vi "60_cm_Scoring.vi"() -> (0 "String":string, 3 "Cluster":cluster{"State":T1, "Drive Control":T2}={"State"=enum."Stop", "Drive Control"={"Left X"=0, "Left Y"=0, "Right Y"=0, "Power (100)"=0, "Wait (ms)"=0, "Enc/Deg Target"=0, "Move Type"=enum."Relative Degrees"}} {"Drive Control"."Power (100)" min=-100 max=100})   [LabVIEW 2012, in "Serenity_mk2.lvrbt"]
uses:
  Serenity_mk2.lvrbt
  State_Typ.ctl
  auto_drive_TYP.ctl
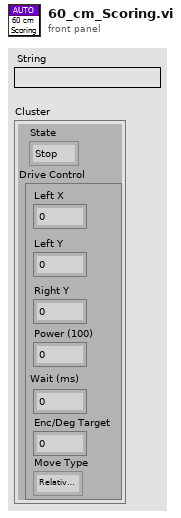
[diagram p1: front panel]
types:
  T1 = typedef "State_Typ.ctl" = enum16{"Sweeper", "Stop", "Check for Position 3", "Check for Position 2", "Move", "Reset Enc", "Read Enc", "Lift", "Dump Close"}
  T2 = typedef "auto_drive_TYP.ctl" = cluster{"Left X":i8, "Left Y":i8, "Right Y":i8, "Power (100)":i8, "Wait (ms)":u32, "Enc/Deg Target":i32, "Move Type":enum16{"Relative Degrees", "Wait", "Encoder"}}
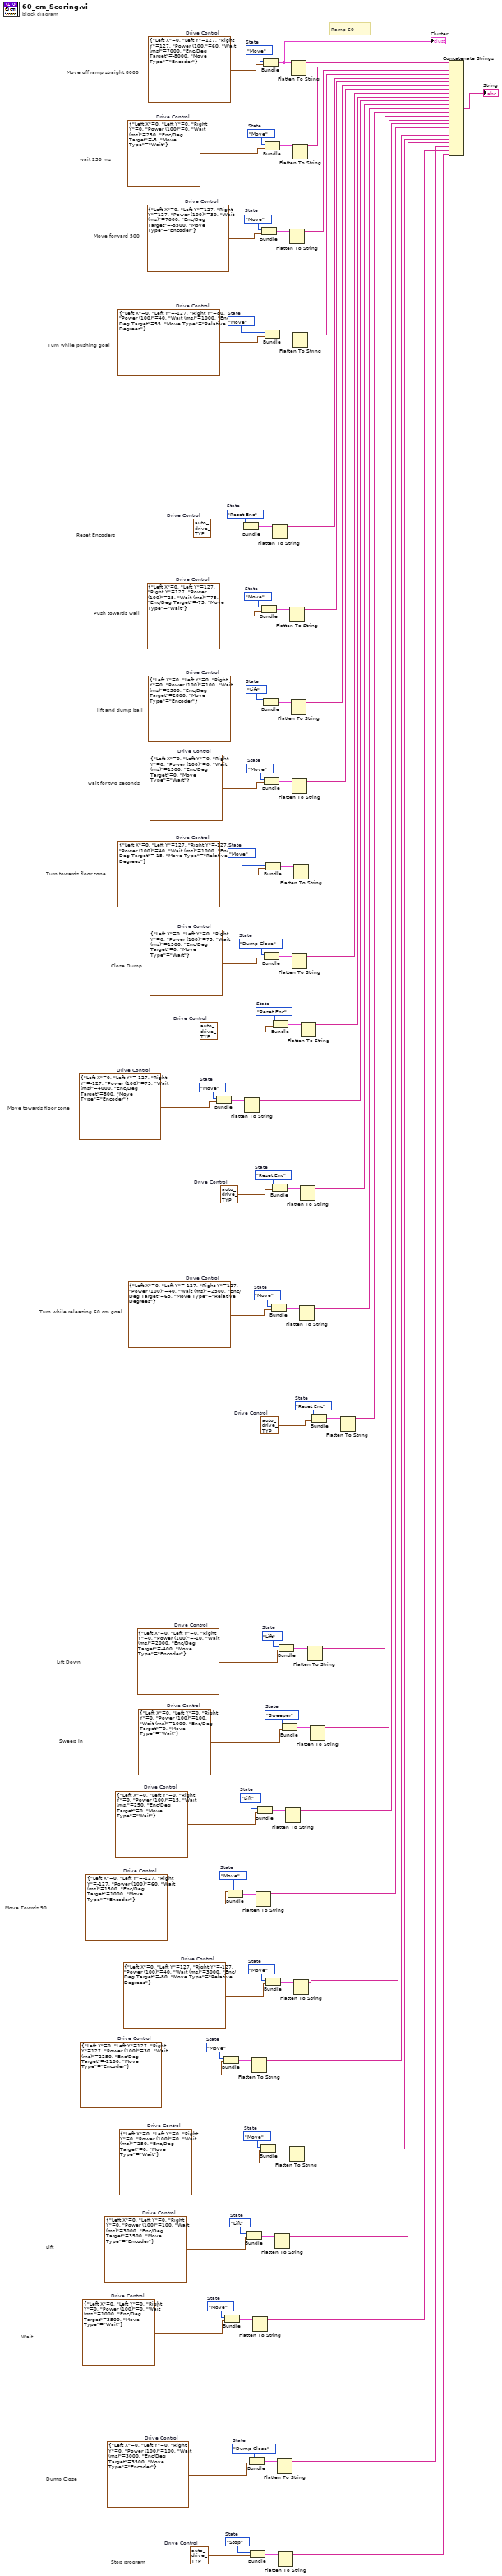
[diagram p0: block diagram]
diagram:
  w5 = T2 {"Left X"=0, "Left Y"=0, "Right Y"=0, "Power (100)"=0, "Wait (ms)"=1000, "Enc/Deg Target"=3500, "Move Type"=enum."Wait"}  # Drive Control
  w3 = State_Typ."Move"  # State
  w8 = T2 {"Left X"=0, "Left Y"=0, "Right Y"=0, "Power (100)"=100, "Wait (ms)"=3000, "Enc/Deg Target"=3500, "Move Type"=enum."Encoder"}  # Drive Control
  w6 = State_Typ."Dump Close"  # State
  w13 = T2 {"Left X"=0, "Left Y"=0, "Right Y"=0, "Power (100)"=100, "Wait (ms)"=3000, "Enc/Deg Target"=3500, "Move Type"=enum."Encoder"}  # Drive Control
  w11 = State_Typ."Lift"  # State
  w16 = T2 {"Left X"=0, "Left Y"=0, "Right Y"=0, "Power (100)"=0, "Wait (ms)"=250, "Enc/Deg Target"=0, "Move Type"=enum."Wait"}  # Drive Control
  w14 = State_Typ."Move"  # State
  w18 = T2 {"Left X"=0, "Left Y"=-127, "Right Y"=50, "Power (100)"=40, "Wait (ms)"=650, "Enc/Deg Target"=-6500, "Move Type"=enum."Wait"}  # Drive Control
  w19 = State_Typ."Reset Enc"  # State
  w27 = T2 {"Left X"=0, "Left Y"=0, "Right Y"=0, "Power (100)"=15, "Wait (ms)"=250, "Enc/Deg Target"=0, "Move Type"=enum."Wait"}  # Drive Control
  w25 = State_Typ."Lift"  # State
  w32 = T2 {"Left X"=0, "Left Y"=0, "Right Y"=0, "Power (100)"=-10, "Wait (ms)"=2000, "Enc/Deg Target"=-400, "Move Type"=enum."Encoder"}  # Drive Control
  w30 = State_Typ."Lift"  # State
  w35 = T2 {"Left X"=0, "Left Y"=0, "Right Y"=0, "Power (100)"=100, "Wait (ms)"=1000, "Enc/Deg Target"=0, "Move Type"=enum."Wait"}  # Drive Control
  w33 = State_Typ."Sweeper"  # State
  w38 = T2 {"Left X"=0, "Left Y"=-127, "Right Y"=-127, "Power (100)"=60, "Wait (ms)"=1500, "Enc/Deg Target"=1000, "Move Type"=enum."Encoder"}  # Drive Control
  w36 = State_Typ."Move"  # State
  w41 = T2 {"Left X"=0, "Left Y"=127, "Right Y"=-127, "Power (100)"=40, "Wait (ms)"=3000, "Enc/Deg Target"=-80, "Move Type"=enum."Relative Degrees"}  # Drive Control
  w39 = State_Typ."Move"  # State
  w46 = T2 {"Left X"=0, "Left Y"=127, "Right Y"=127, "Power (100)"=30, "Wait (ms)"=2250, "Enc/Deg Target"=-2100, "Move Type"=enum."Encoder"}  # Drive Control
  w44 = State_Typ."Move"  # State
  w51 = T2 {"Left X"=0, "Left Y"=127, "Right Y"=127, "Power (100)"=20, "Wait (ms)"=7000, "Enc/Deg Target"=-8500, "Move Type"=enum."Encoder"}  # Drive Control
  w50 = State_Typ."Reset Enc"  # State
  w54 = T2 {"Left X"=0, "Left Y"=127, "Right Y"=127, "Power (100)"=25, "Wait (ms)"=75, "Enc/Deg Target"=-75, "Move Type"=enum."Wait"}  # Drive Control
  w53 = State_Typ."Move"  # State
  w58 = T2 {"Left X"=0, "Left Y"=0, "Right Y"=0, "Power (100)"=50, "Wait (ms)"=4000, "Enc/Deg Target"=-9000, "Move Type"=enum."Encoder"}  # Drive Control
  w59 = State_Typ."Reset Enc"  # State
  w61 = T2 {"Left X"=0, "Left Y"=-127, "Right Y"=-127, "Power (100)"=75, "Wait (ms)"=4000, "Enc/Deg Target"=800, "Move Type"=enum."Encoder"}  # Drive Control
  w62 = State_Typ."Move"  # State
  w65 = T2 {"Left X"=0, "Left Y"=-127, "Right Y"=80, "Power (100)"=40, "Wait (ms)"=1000, "Enc/Deg Target"=55, "Move Type"=enum."Relative Degrees"}  # Drive Control
  w66 = State_Typ."Move"  # State
  w69 = T2 {"Left X"=0, "Left Y"=0, "Right Y"=0, "Power (100)"=0, "Wait (ms)"=250, "Enc/Deg Target"=-5, "Move Type"=enum."Wait"}  # Drive Control
  w70 = State_Typ."Move"  # State
  w73 = T2 {"Left X"=0, "Left Y"=127, "Right Y"=127, "Power (100)"=30, "Wait (ms)"=7000, "Enc/Deg Target"=-8500, "Move Type"=enum."Encoder"}  # Drive Control
  w74 = State_Typ."Move"  # State
  w78 = T2 {"Left X"=0, "Left Y"=0, "Right Y"=0, "Power (100)"=75, "Wait (ms)"=1500, "Enc/Deg Target"=0, "Move Type"=enum."Wait"}  # Drive Control
  w79 = State_Typ."Dump Close"  # State
  w101 = T2 {"Left X"=0, "Left Y"=0, "Right Y"=0, "Power (100)"=0, "Wait (ms)"=1500, "Enc/Deg Target"=0, "Move Type"=enum."Wait"}  # Drive Control
  w102 = State_Typ."Move"  # State
  w98 = T2 {"Left X"=0, "Left Y"=-127, "Right Y"=50, "Power (100)"=40, "Wait (ms)"=650, "Enc/Deg Target"=-6500, "Move Type"=enum."Wait"}  # Drive Control
  w99 = State_Typ."Reset Enc"  # State
  w95 = T2 {"Left X"=0, "Left Y"=-127, "Right Y"=127, "Power (100)"=40, "Wait (ms)"=2500, "Enc/Deg Target"=65, "Move Type"=enum."Relative Degrees"}  # Drive Control
  w96 = State_Typ."Move"  # State
  w85 = T2 {"Left X"=0, "Left Y"=0, "Right Y"=-127, "Power (100)"=40, "Wait (ms)"=700, "Enc/Deg Target"=-6500, "Move Type"=enum."Wait"}  # Drive Control
  w92 = T2 {"Left X"=0, "Left Y"=127, "Right Y"=-127, "Power (100)"=40, "Wait (ms)"=1000, "Enc/Deg Target"=-15, "Move Type"=enum."Relative Degrees"}  # Drive Control
  w93 = State_Typ."Move"  # State
  w90 = T2 {"Left X"=0, "Left Y"=0, "Right Y"=0, "Power (100)"=100, "Wait (ms)"=2500, "Enc/Deg Target"=2800, "Move Type"=enum."Encoder"}  # Drive Control
  w89 = State_Typ."Lift"  # State
  w86 = State_Typ."Stop"  # State
  w81 = T2 {"Left X"=0, "Left Y"=127, "Right Y"=127, "Power (100)"=60, "Wait (ms)"=7000, "Enc/Deg Target"=-8000, "Move Type"=enum."Encoder"}  # Drive Control
  w82 = State_Typ."Move"  # State
  # "Wait"
  # "Dump Close"
  # "Lift"
  # "Lift Down"
  # "Sweep In"
  # "Move Towrds 90"
  # "Reset Encoders"
  # "Push towards wall"
  # "Stop program"
  # "Turn while releasing 60 cm goal"
  # "Move towards floor zone"
  # "Close Dump"
  # "Turn towards floor zone"
  # "Move forward 500"
  # "Turn while pushing goal"
  # "lift and dump ball"
  # "wait 250 ms"
  # "wait for two seconds"
  # "Move off ramp straight 8000"
  # "Ramp 60"
  n1 = Bundle("State"=w62, "Drive Control"=w61) -> (w63:cluster{"State":T1, "Drive Control":T2})  [unwired: 1 in]
  n2 = Bundle("State"=w44, "Drive Control"=w46) -> (w45:cluster{"State":T1, "Drive Control":T2})  [unwired: 1 in]
  n3 = Bundle("State"=w3, "Drive Control"=w5) -> (w4:cluster{"State":T1, "Drive Control":T2})  [unwired: 1 in]
  n4 = Bundle("State"=w36, "Drive Control"=w38) -> (w37:cluster{"State":T1, "Drive Control":T2})  [unwired: 1 in]
  n5 = Bundle("State"=w50, "Drive Control"=w51) -> (w49:cluster{"State":T1, "Drive Control":T2})  [unwired: 1 in]
  n6 = Flatten To String(anything=w63) -> (data string=w55:string)  [unwired: 3 in, 2 out]
  n7 = Bundle("State"=w11, "Drive Control"=w13) -> (w12:cluster{"State":T1, "Drive Control":T2})  [unwired: 1 in]
  n8 = Bundle("State"=w6, "Drive Control"=w8) -> (w7:cluster{"State":T1, "Drive Control":T2})  [unwired: 1 in]
  n9 = Bundle("State"=w86, "Drive Control"=w85) -> (w87:cluster{"State":T1, "Drive Control":T2})  [unwired: 1 in]
  n10 = Flatten To String(anything=w45) -> (data string=w22:string)  [unwired: 3 in, 2 out]
  n11 = Flatten To String(anything=w4) -> (data string=w1:string)  [unwired: 3 in, 2 out]
  n12 = Flatten To String(anything=w37) -> (data string=w23:string)  [unwired: 3 in, 2 out]
  n13 = Bundle("State"=w25, "Drive Control"=w27) -> (w26:cluster{"State":T1, "Drive Control":T2})  [unwired: 1 in]
  n14 = Bundle("State"=w14, "Drive Control"=w16) -> (w15:cluster{"State":T1, "Drive Control":T2})  [unwired: 1 in]
  n15 = Bundle("State"=w74, "Drive Control"=w73) -> (w75:cluster{"State":T1, "Drive Control":T2})  [unwired: 1 in]
  n16 = Bundle("State"=w53, "Drive Control"=w54) -> (w52:cluster{"State":T1, "Drive Control":T2})  [unwired: 1 in]
  n17 = Bundle("State"=w82, "Drive Control"=w81) -> (w83:cluster{"State":T1, "Drive Control":T2})  [unwired: 1 in]
  "Cluster" <- w83
  n18 = Bundle("State"=w89, "Drive Control"=w90) -> (w88:cluster{"State":T1, "Drive Control":T2})  [unwired: 1 in]
  n19 = Bundle("State"=w102, "Drive Control"=w101) -> (w103:cluster{"State":T1, "Drive Control":T2})  [unwired: 1 in]
  n20 = Bundle("State"=w79, "Drive Control"=w78) -> (w80:cluster{"State":T1, "Drive Control":T2})  [unwired: 1 in]
  n21 = Bundle("State"=w70, "Drive Control"=w69) -> (w71:cluster{"State":T1, "Drive Control":T2})  [unwired: 1 in]
  n22 = Bundle("State"=w66, "Drive Control"=w65) -> (w67:cluster{"State":T1, "Drive Control":T2})  [unwired: 1 in]
  n23 = Bundle("State"=w93, "Drive Control"=w92) -> (w94:cluster{"State":T1, "Drive Control":T2})  [unwired: 1 in]
  n24 = Bundle("State"=w39, "Drive Control"=w41) -> (w40:cluster{"State":T1, "Drive Control":T2})  [unwired: 1 in]
  n25 = Bundle("State"=w96, "Drive Control"=w95) -> (w97:cluster{"State":T1, "Drive Control":T2})  [unwired: 1 in]
  n26 = Flatten To String(anything=w49) -> (data string=w48:string)  [unwired: 3 in, 2 out]
  n27 = Bundle("State"=w99, "Drive Control"=w98) -> (w100:cluster{"State":T1, "Drive Control":T2})  [unwired: 1 in]
  n28 = Bundle("State"=w59, "Drive Control"=w58) -> (w60:cluster{"State":T1, "Drive Control":T2})  [unwired: 1 in]
  n29 = Flatten To String(anything=w12) -> (data string=w9:string)  [unwired: 3 in, 2 out]
  n30 = Flatten To String(anything=w7) -> (data string=w2:string)  [unwired: 3 in, 2 out]
  n31 = Flatten To String(anything=w87) -> (data string=w43:string)  [unwired: 3 in, 2 out]
  n32 = Bundle("State"=w30, "Drive Control"=w32) -> (w31:cluster{"State":T1, "Drive Control":T2})  [unwired: 1 in]
  n33 = Bundle("State"=w33, "Drive Control"=w35) -> (w34:cluster{"State":T1, "Drive Control":T2})  [unwired: 1 in]
  n34 = Flatten To String(anything=w26) -> (data string=w24:string)  [unwired: 3 in, 2 out]
  n35 = Flatten To String(anything=w15) -> (data string=w10:string)  [unwired: 3 in, 2 out]
  n36 = Flatten To String(anything=w75) -> (data string=w72:string)  [unwired: 3 in, 2 out]
  n37 = Flatten To String(anything=w52) -> (data string=w47:string)  [unwired: 3 in, 2 out]
  n38 = Flatten To String(anything=w83) -> (data string=w76:string)  [unwired: 3 in, 2 out]
  n39 = Flatten To String(anything=w88) -> (data string=w91:string)  [unwired: 3 in, 2 out]
  n40 = Flatten To String(anything=w103) -> (data string=w104:string)  [unwired: 3 in, 2 out]
  n41 = Flatten To String(anything=w80) -> (data string=w77:string)  [unwired: 3 in, 2 out]
  n42 = Flatten To String(anything=w71) -> (data string=w68:string)  [unwired: 3 in, 2 out]
  n43 = Flatten To String(anything=w67) -> (data string=w64:string)  [unwired: 3 in, 2 out]
  n44 = Flatten To String(anything=w94) -> ()  [unwired: 3 in, 3 out]
  n45 = Flatten To String(anything=w40) -> (data string=w21:string)  [unwired: 3 in, 2 out]
  n46 = Flatten To String(anything=w97) -> (data string=w42:string)  [unwired: 3 in, 2 out]
  n47 = Flatten To String(anything=w100) -> (data string=w56:string)  [unwired: 3 in, 2 out]
  n48 = Flatten To String(anything=w60) -> (data string=w57:string)  [unwired: 3 in, 2 out]
  n49 = Flatten To String(anything=w31) -> (data string=w28:string)  [unwired: 3 in, 2 out]
  n50 = Flatten To String(anything=w34) -> (data string=w29:string)  [unwired: 3 in, 2 out]
  n51 = Bundle("State"=w19, "Drive Control"=w18) -> (w20:cluster{"State":T1, "Drive Control":T2})  [unwired: 1 in]
  n52 = Flatten To String(anything=w20) -> (data string=w17:string)  [unwired: 3 in, 2 out]
  n53 = Concatenate Strings(w76, w68, w72, w64, w48, w47, w91, w104, w77, w57, w55, w56, w42, w17, w28, w29, w24, w23, w21, w22, w10, w9, w1, w2, w43) -> (→"String":string)
